vi "SOAE-Add Plot.vi"(0 "Graph":refnum<vi>, 5 "Listbox":refnum<vi>, 7 "Path in":path, 9 "XY Data":cluster{dbl[], dbl[]}={[nan], [nan]}) -> (8 "Path out":path)   [LabVIEW 2020]
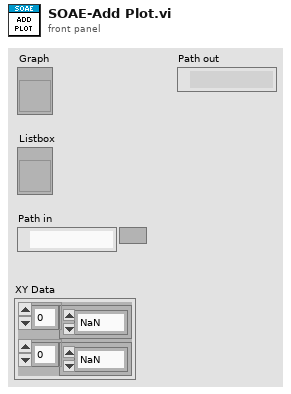
[diagram p1: front panel]
types:
  T1 = enum16{"User", "Prism", "Kelly", "Dark2", "Sequential", "Hue"}
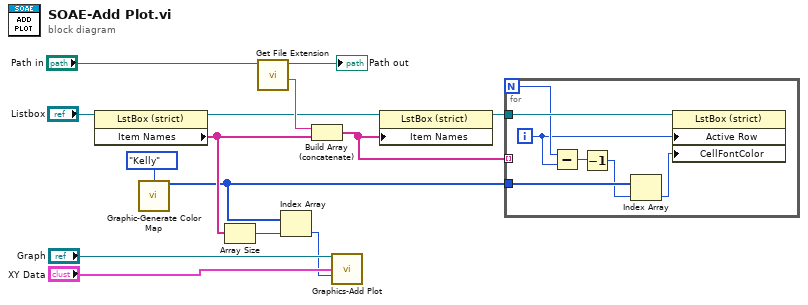
[diagram p0: block diagram]
diagram:
  n1 = property class="LstBox (strict)"(reference="Listbox") -> (reference out=w4:refnum<vi>, "Item Names"=w8:string[])  [unwired: 1 in, 1 out]
  n2 = call "Graphic-Generate Color Map.vi"("Map"=T1."Kelly") -> ("Colors"=w1:u32[])  [unwired: 14 in]
  n3 = Array Size(array=w8) -> (size(s)=w10:i32)
  n4 = call <vilib>:"Get File Extension.vi"("file"="Path in") -> ("filename without extension"=w5:string, "dup file"=→"Path out":path)  [unwired: 6 in, 3 out]
  n5 = Index Array(array=w1, index=w10) -> (element=w9:u32)
  n6 = Build Array (concatenate)(w5, w8) -> (w2:string[])
  n7 = call "Graphics-Add Plot.vi"("XYGraph in"="Graph", "XY Data"="XY Data", "Color"=w9) -> ()  [unwired: 11 in, 2 out]
  n8 = property class="LstBox (strict)"(reference=w4, "Item Names"=w2) -> (reference out=w3:refnum<vi>)  [unwired: 1 in, 1 out]
  n9 = for {
    N -> [w19]
    tunnel: w3 -> [w21]
    tunnel: w2 -> [_] mode=indexing
    tunnel: w1 -> [w20]
    i -> [w17]
    n10 = Subtract(x=w19, y=w17) -> (x-y=w18:i32)
    n11 = Decrement(x=w18) -> (x-1=w16:i32)
    n12 = Index Array(array=w20, index=w16) -> (element=w15:u32)
    n13 = property class="LstBox (strict)"(reference=w21, "Active Row"=w17, "CellFontColor"=w15) -> ()  [unwired: 1 in, 2 out]
  }
